vi "test.crc32.vi"() -> (3 "All Passed":bool)   [LabVIEW 2020]
uses:
  Market.Data.Common/fpga/my.network.data.stream.ctl
  crc.test.case.ctl
  Market.Data.Bats.Parser/fpga/data.ctl
panel:
  in  "Test #":i16=10
  in  "Override":bool
  in  "Test Case #1 - Buffer is Empty, Data has 8 elements":T1={"data.valid"=TRUE, "buffer"=[0, 0, 0, 0, 0, 0, 0, 0, 0], "buffer.length"=0, "exp.buffer.value.1"=1234605616436508552, "index 1"=0, "exp.buffer.value.2"=0, "index 2"=1, "exp.buffer.length"=8, "Key (U64)"=0, "data"={"enabled"=[TRUE, TRUE, TRUE, TRUE, TRUE, TRUE, TRUE, TRUE], "byte"=[17, 34, 51, 68, 85, 102, 119, 136]}} {"data"."byte" format="%.0x"; "index 2" format="%.0x"; "exp.buffer.value.2" format="%.0x"; "index 1" format="%.0x"; "exp.buffer.value.1" format="%.0x"; "buffer" format="%.0x"}
  out "Passed 1":bool
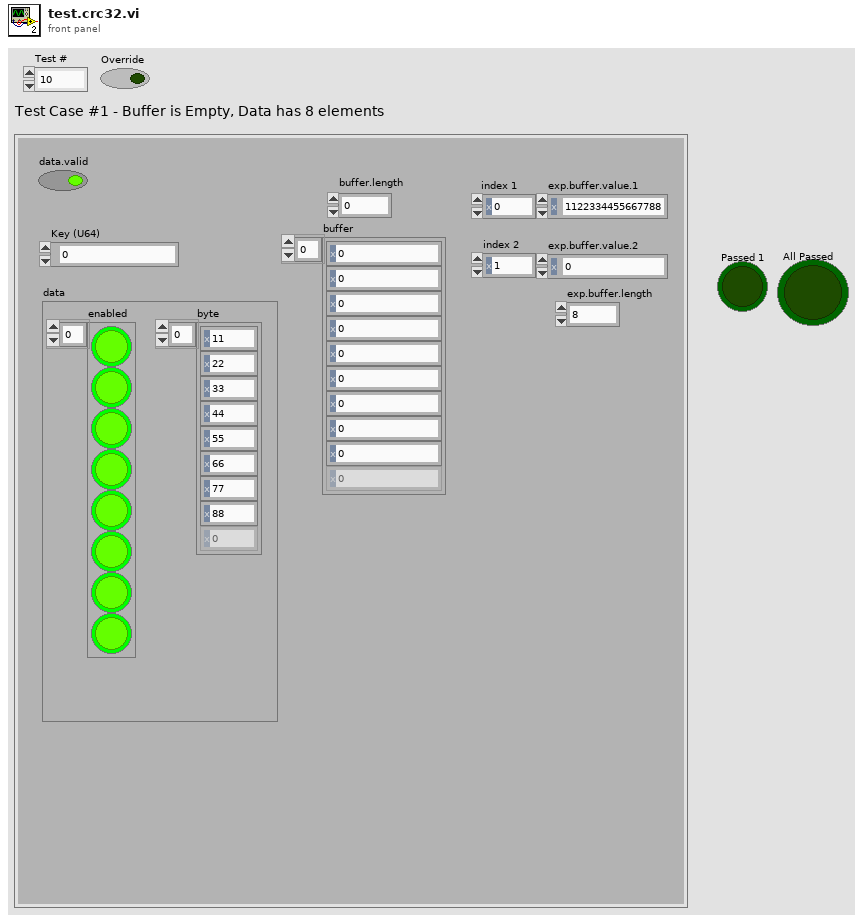
[diagram p1: front panel]
types:
  T1 = typedef "crc.test.case.ctl" = cluster{"data.valid":bool, "buffer":u64[], "buffer.length":u8, "exp.buffer.value.1":u64, "index 1":i16, "exp.buffer.value.2":u64, "index 2":i16, "exp.buffer.length":u8, "Key (U64)":u64, "data":T2}
  T2 = typedef "data.ctl" = cluster{"enabled":bool[], "byte":u8[]}
  T3 = typedef "my.network.data.stream.ctl" = cluster{"data":u8[], "data valid":bool, "byte enables":bool[], "eof.good":bool, "eof.bad":bool, "Timestamp":u64}
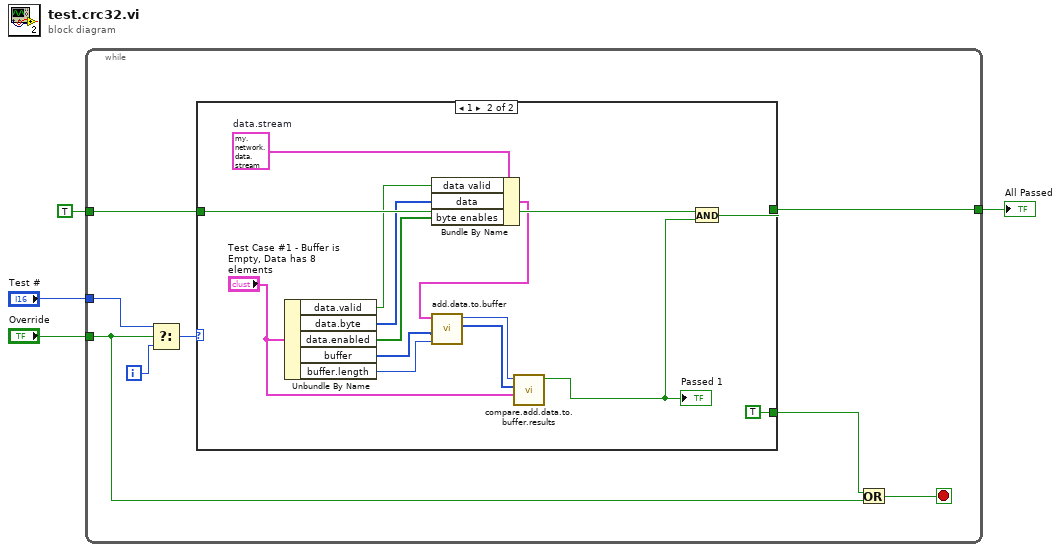
[diagram p0: block diagram]
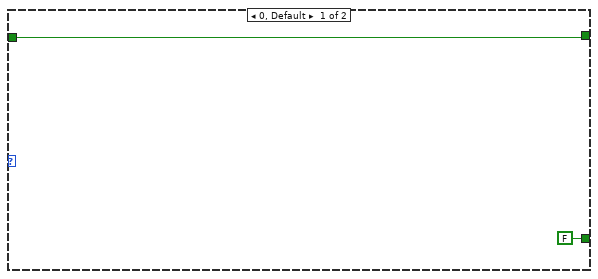
[diagram p2: hidden frame]
diagram:
  n1 = while {
    tunnel: TRUE -> [w11]
    tunnel: [w10] -> w3
    tunnel: "Test #" -> [w9]
    tunnel: "Override" -> [w5]
    i -> [w8]
    stop <- w6 stop-if-true
    n2 = Select(t=w9, s=w5, f=w8) -> (s? t:f=w7:i32)
    n3 = case shown="1" w7 {
      tunnel: [FALSE TRUE] -> w12
      tunnel: w11 -> [w14 w22]
      tunnel: [w14 w24] -> w10
      frame 0, Default {
      }
      frame 1 {
        w21 = T3 {"data"=[0, 0, 0, 0, 0, 0, 0, 0], "data valid"=FALSE, "byte enables"=[FALSE, FALSE, FALSE, FALSE, FALSE, FALSE, FALSE, FALSE], "eof.good"=FALSE, "eof.bad"=FALSE, "Timestamp"=0}  # data.stream
        n4 = Unbundle By Name("Test Case #1 - Buffer is Empty, Data has 8 elements") -> ("data.valid"=w20:bool, "data.byte"=w19:u8[], "data.enabled"=w15:bool[], "buffer"=w26:u64[], "buffer.length"=w25:u8)
        n5 = Bundle By Name(cluster=w21, "data valid"=w20, "data"=w19, "byte enables"=w15) -> (w18:T3)
        n6 = call "add.data.to.buffer.vi"("buffer.length"=w25, "buffer"=w26, "data.stream"=w18) -> ("buffer.out"=w27:u64[], "buffer.length.out"=w28:u8)  [unwired: 7 in]
        n7 = call "compare.add.data.to.buffer.results.vi"("Test Case"="Test Case #1 - Buffer is Empty, Data has 8 elements", "buffer.out"=w27, "buffer.length.out"=w28) -> ("All Passed"=w23:bool)  [unwired: 8 in]
        "Passed 1" <- w23
        n8 = And(x=w22, y=w23) -> (x .and. y?=w24:bool)
      }
    }
    n9 = Or(x=w12, y=w5) -> (x .or. y?=w6:bool)
  }
  "All Passed" <- w3
